vi "Set Titles.vi"(8 "error in (no error)":errorcluster, 10 "Titles":string[](array[string]), 11 "List in":refnum<class "List.lvclass">) -> (0 "error out":errorcluster, 3 "List out":refnum<class "List.lvclass">)   [LabVIEW 2015, in "List.lvclass"]
uses:
  List.lvclass
  List.lvclass/List.ctl
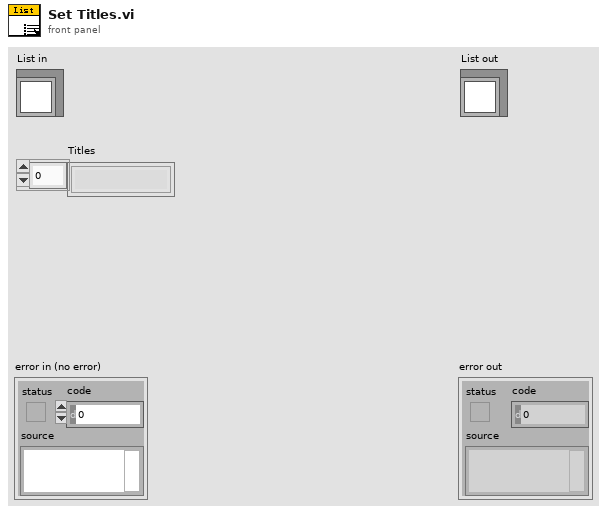
[diagram p1: front panel]
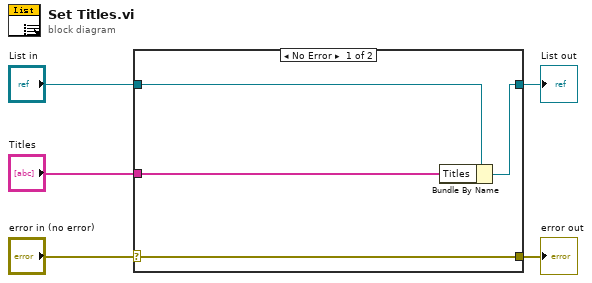
[diagram p0: block diagram]
diagram:
  n1 = case shown="No Error" "error in (no error)" {
    selector: "error in (no error)" -> [w9 w10]
    tunnel: [w9 w10] -> w4
    tunnel: [w7 w11] -> w2
    tunnel: "List in" -> [w8 w11]
    tunnel: "Titles" -> [w6 _]
    frame No Error {
      n2 = Bundle By Name(cluster=w8, "Titles"=w6) -> (w7:refnum<class "List.lvclass">)
    }
    frame Error {
    }
  }
  "error out" <- w4
  "List out" <- w2
